vi "1.vi"(8 "error in (no error)":errorcluster, 10 "adat":T1) -> (0 "error out":errorcluster, 2 "adat":T1, 3 "Waveform Graph":dbl[][](graph), 4 "XY Graph":cluster{dbl[], "yi":dbl[]}[](graph))   [LabVIEW 2016]
doc: "Fájlbeolvasás, ablakolás, lineáris interpoláció."
uses:
  adat.ctl
  <vilib>/Utility/file.llb/Read Delimited Spreadsheet (DBL).vi
  <vilib>/gmath/NI_Gmath.lvlib
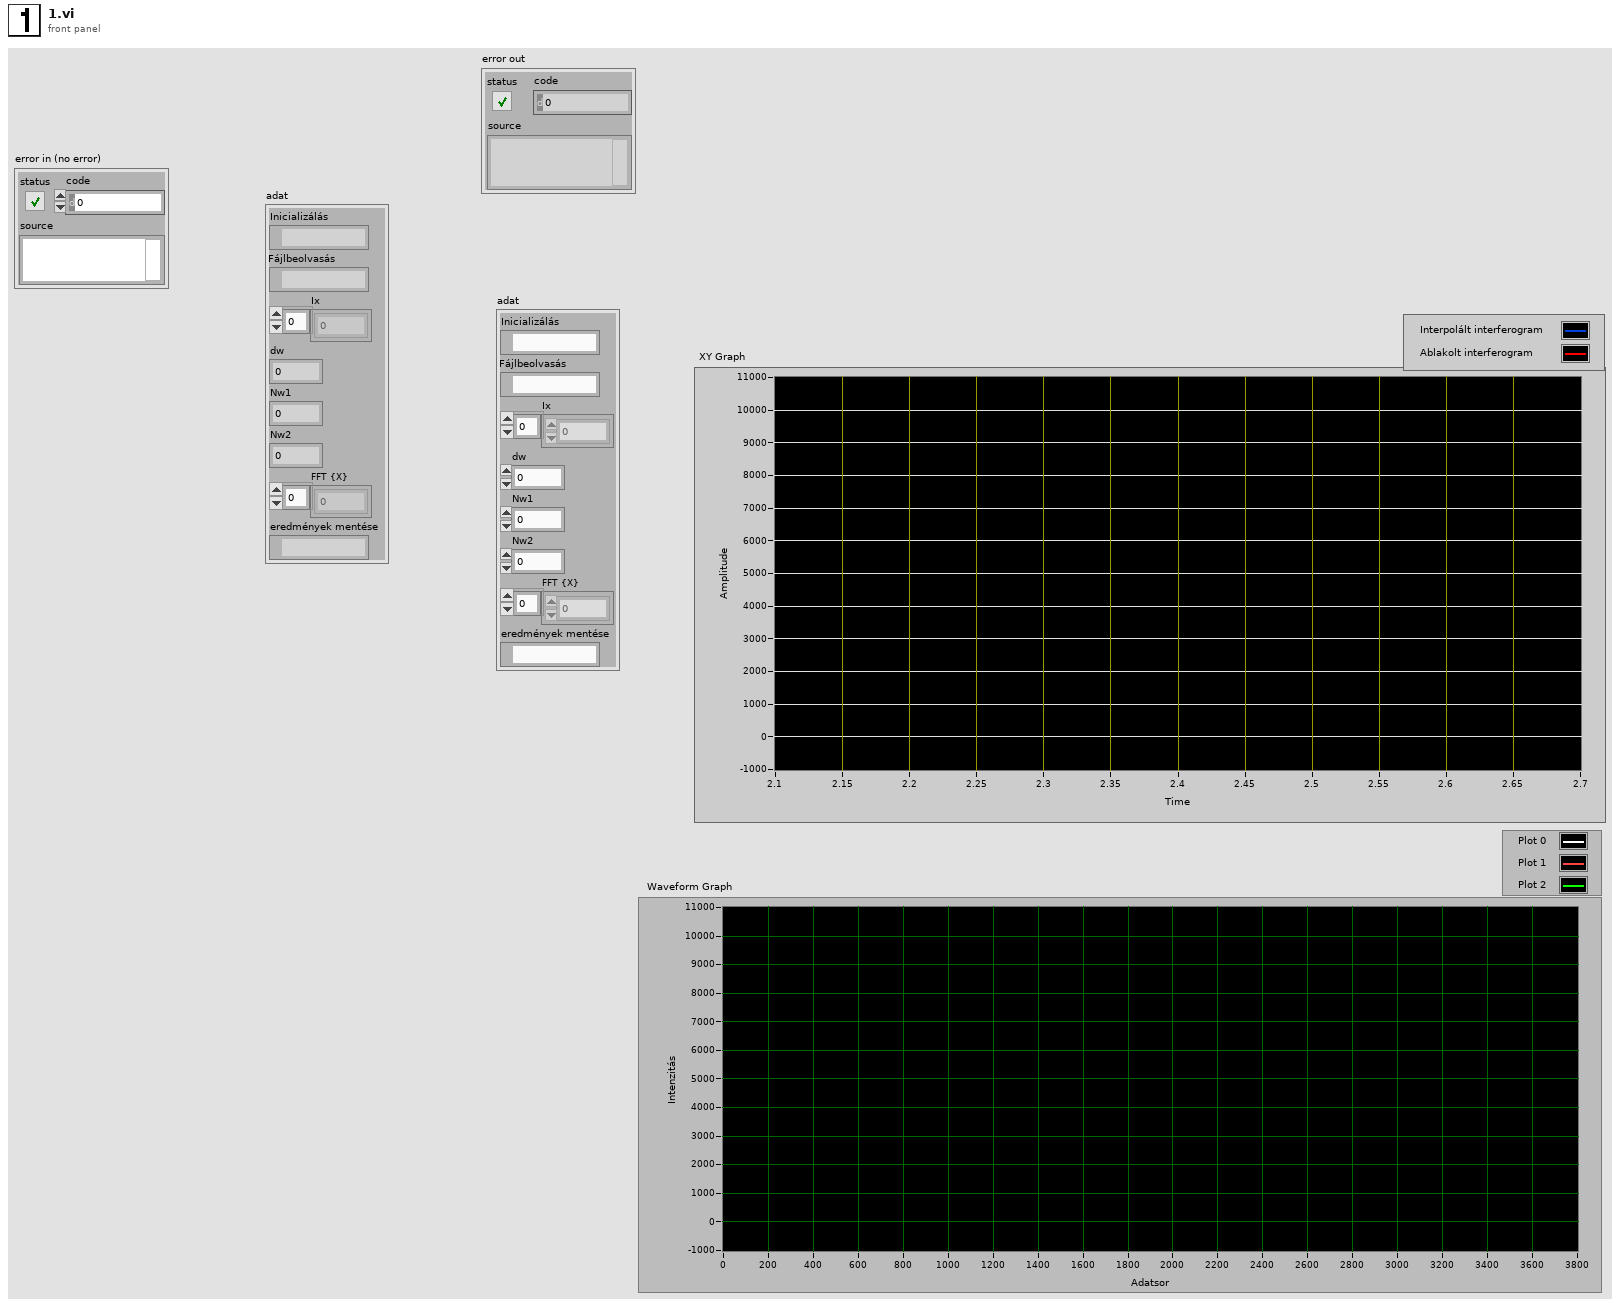
[diagram p1: front panel]
types:
  T1 = typedef "adat.ctl" = cluster{"Inicializálás":path, "Fájlbeolvasás":path, "Ix":dbl[], "dw":dbl, "Nw1":dbl, "Nw2":dbl, "FFT {X}":cdb[], "eredmények mentése":path}
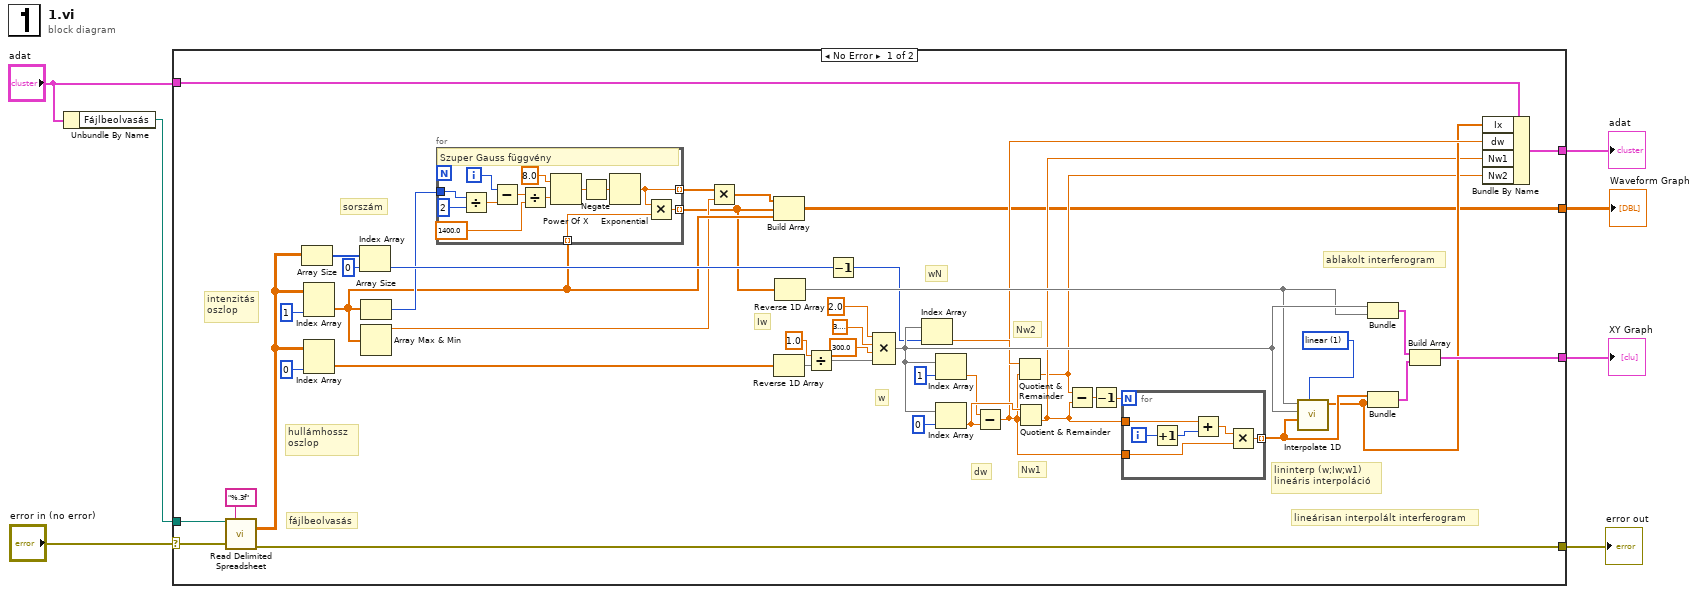
[diagram p0: block diagram]
diagram:
  n1 = Unbundle By Name("adat") -> ("Fájlbeolvasás"=w4:path)
  n2 = case shown="No Error" "error in (no error)" {
    selector: "error in (no error)" -> [w22 w72]
    tunnel: w4 -> [w28 _]
    tunnel: [w23 _] -> w7
    tunnel: "adat" -> [w21 w73]
    tunnel: [w16 w73] -> w6
    tunnel: [w15 w72] -> w2
    tunnel: [w13 _] -> w1
    frame No Error {
      w52 = 1 items=["nearest", "linear", "spline", "cubic Hermite", "Lagrange"] ("method")
      # "fájlbeolvasás"
      # "ablakolt interferogram"
      # "lineárisan interpolált interferogram"
      # "wN"
      # "dw"
      # "lininterp (w;Iw;w1)\nlineáris interpoláció"
      # "w"
      # "Nw2"
      # "Nw1"
      # "Iw"
      # "intenzitás\noszlop"
      # "hullámhossz \noszlop"
      # "sorszám"
      n3 = call-poly <vilib>:"Read Delimited Spreadsheet.vi"("file path (dialog if empty)"=w28, "format (%.3f)"="%.3f", "error in (no error)"=w22) -> ("all rows"=w32:dbl[][], "error out"=w15:errorcluster)  [unwired: 7 in, 4 out]
      n4 = Array Size(array=w32) -> (size(s)=w26:i32[])
      n5 = Index Array(array=w32, index (col)=1 ("disabled index (col)")) -> (element=w12:dbl[])  [unwired: 1 in]
      n6 = Index Array(array=w32, index (col)=0 ("disabled index (col)")) -> (element=w30:dbl[])  [unwired: 1 in]
      n7 = Index Array(array=w26, index=0) -> (element=w27:i32)
      n8 = Array Size(array=w12) -> (size(s)=w14:i32)
      n9 = Array Max & Min(array=w12) -> (max value=w11:dbl)  [unwired: 3 out]
      n10 = for {
        tunnel: w14 -> [w65]
        tunnel: w12 -> [w57] mode=indexing
        tunnel: [w56] -> w8 mode=indexing
        tunnel: [w53] -> w10 mode=indexing
        i -> [w62]
        # "Szuper Gauss függvény"
        n11 = Divide(x=w65, y=2) -> (x/y=w63:dbl)
        n12 = Subtract(x=w62, y=w63) -> (x-y=w61:dbl)
        n13 = Divide(x=w61, y=1400.0) -> (x/y=w59:dbl)
        n14 = Power Of X(1:w59, 2:8.0 ("y")) -> (0:w55:dbl)
        n15 = Negate(x=w55) -> (-x=w54:dbl)
        n16 = Exponential(1:w54) -> (0:w53:dbl)
        n17 = Multiply(x=w53, y=w57) -> (x*y=w56:dbl)
      }
      n18 = Multiply(x=w10, y=w11) -> (x*y=w9:dbl[])
      n19 = Build Array(w9, w8, w12) -> (w13:dbl[][])
      n20 = Reverse 1D Array(array=w30) -> (reversed array=w38:dbl[])
      n21 = Reverse 1D Array(array=w8) -> (reversed array=w46:dbl[])
      n22 = Divide(x=1.0, y=w38) -> (x/y=w39:dbl[])
      n23 = Decrement(x=w27) -> (x-1=w43:i32)
      n24 = Compound Arithmetic op=MULTIPLY(2.0 ("value"), 3.141592653589793, 300.0 ("value"), w39) -> (w47:dbl[])
      n25 = Index Array(array=w47, index=w43) -> (element=w44:dbl)
      n26 = Index Array(array=w47, index=1) -> (element=w42:dbl)
      n27 = Index Array(array=w47, index=0) -> (element=w45:dbl)
      n28 = Subtract(x=w42, y=w45) -> (x-y=w20:dbl)
      n29 = Quotient & Remainder(x=w44, y=w20) -> (floor(x/y)=w17:dbl)  [unwired: 1 out]
      n30 = Quotient & Remainder(x=w45, y=w20) -> (floor(x/y)=w18:dbl)  [unwired: 1 out]
      n31 = Subtract(x=w17, y=w18) -> (x-y=w37:dbl)
      n32 = Decrement(x=w37) -> (x-1=w48:dbl)
      n33 = for {
        N: w48 -> [_]
        tunnel: w18 -> [w70]
        tunnel: w20 -> [w66]
        tunnel: [w69] -> w49 mode=indexing
        i -> [w68]
        n34 = Increment(x=w68) -> (x+1=w71:i32)
        n35 = Add(x=w70, y=w71) -> (x+y=w67:dbl)
        n36 = Multiply(x=w67, y=w66) -> (x*y=w69:dbl)
      }
      n37 = call <vilib>:"Interpolate 1D.vi"("method"=w52, "xi"=w49, "X"=w47, "Y"=w46) -> ("yi"=w19:dbl[])  [unwired: 5 in, 2 out]
      n38 = Bundle(w47, w46) -> (w50:cluster{dbl[], dbl[]})  [unwired: 1 in]
      n39 = Bundle(w49, "yi"=w19) -> (w51:cluster{dbl[], "yi":dbl[]})  [unwired: 1 in]
      n40 = Build Array(w50, w51) -> (w23:cluster{dbl[], "yi":dbl[]}[])
      n41 = Bundle By Name(cluster=w21, "Ix"=w19, "dw"=w20, "Nw1"=w18, "Nw2"=w17) -> (w16:T1)
    }
    frame Error {
    }
  }
  "XY Graph" <- w7
  "error out" <- w2
  "adat" <- w6
  "Waveform Graph" <- w1
